vi "Get_MEAN_A+Phi.vi"(5 "Frequency [Hz]":dbl, 6 "error in (no error)":errorcluster) -> (0 "Mean Amplitude":dbl, 1 "Error Amplitude":dbl, 2 "Mean Phase Shift":dbl, 3 "error out":errorcluster, 4 "Error Phase Shift":dbl)   [LabVIEW 2010]
panel:
  in  "Wait [s]":dbl=0.5
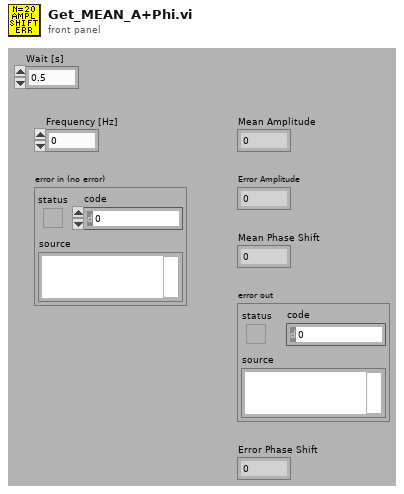
[diagram p1: front panel]
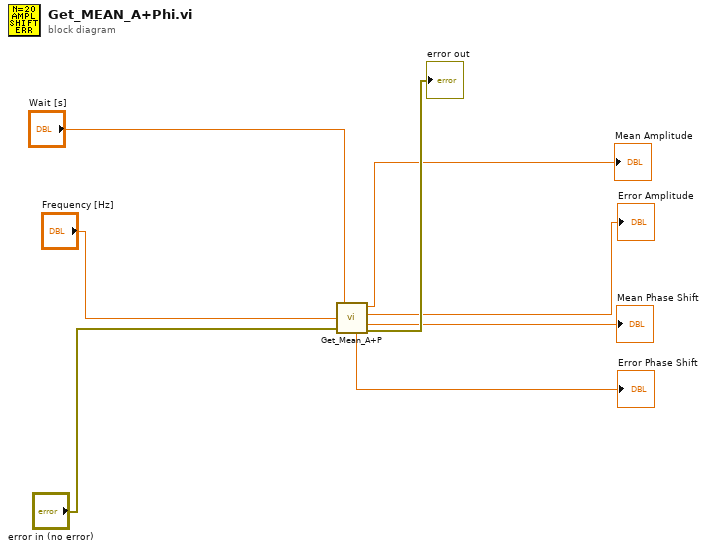
[diagram p0: block diagram]
diagram:
  n1 = call "Get_Mean_A+P.vi"("Wait"="Wait [s]", "Frequency"="Frequency [Hz]", "error in (no error)"="error in (no error)") -> ("Mean Amplitude"=→"Mean Amplitude":dbl, "Error Amplitude"=→"Error Amplitude":dbl, "Mean Phase Shift"=→"Mean Phase Shift":dbl, "error out"=→"error out":errorcluster, "Error Phase Shift"=→"Error Phase Shift":dbl)
